vi "RW Cutoff Array.vi"(0 "Refnum In":T1, 2 "Read (F)":bool, 7 "CutoffArray In":cluster{"MidCutoff":dbl, "CloseCutoff":dbl}[](array[cluster]), 11 "Error In":errorcluster) -> (4 "Refnum Out":T1, 8 "CutoffArray Out":cluster{"MidCutoff":dbl, "CloseCutoff":dbl}[](array[cluster]), 15 "Error Out":errorcluster)   [LabVIEW 2013]
uses:
  <vilib>/Utility/config.llb/Config Data RefNum.ctl
  <vilib>/Utility/config.llb/Write Key (Double).vi
  <vilib>/Utility/config.llb/Read Key (Double).vi
  <vilib>/Utility/config.llb/NI_LVConfig.lvlib
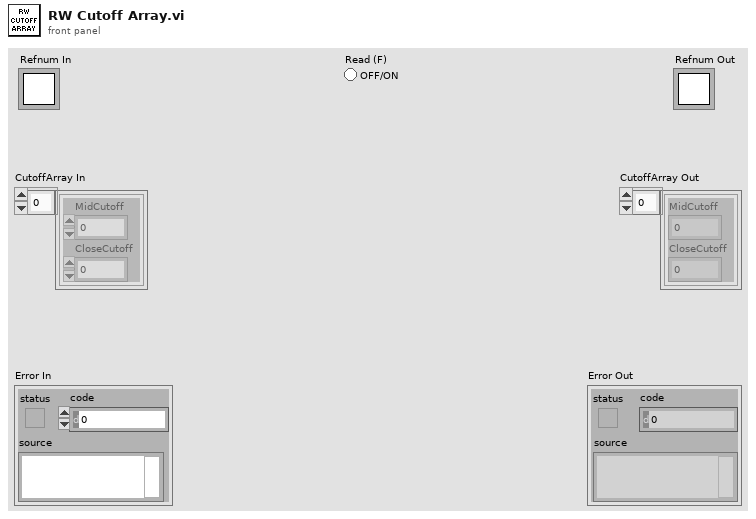
[diagram p1: front panel]
types:
  T1 = typedef "NI_LVConfig.lvlib/Config Data RefNum.ctl" = refnum<k1>
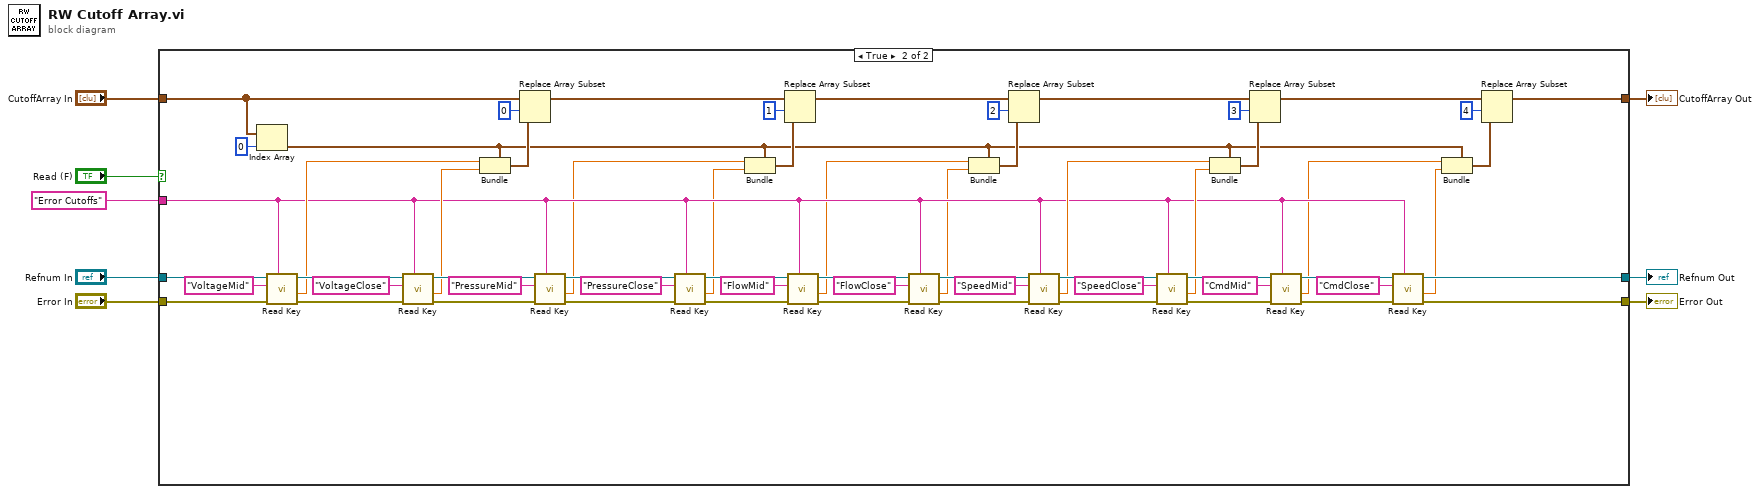
[diagram p0: block diagram]
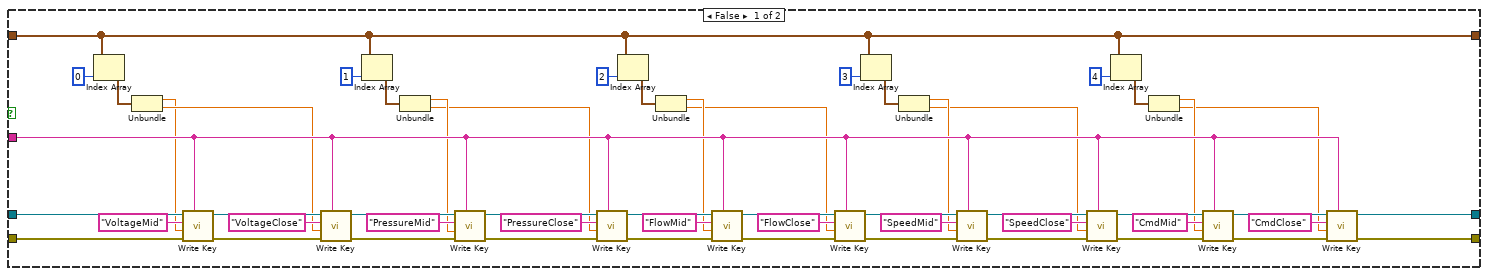
[diagram p2: hidden frame]
diagram:
  n1 = case shown="True" "Read (F)" {
    tunnel: "Error In" -> [w62 w122]
    tunnel: [w25 w89] -> w7
    tunnel: "Refnum In" -> [w53 w123]
    tunnel: [w26 w90] -> w4
    tunnel: "Error Cutoffs" ("section") -> [w24 w78]
    tunnel: "CutoffArray In" -> [w19 w104]
    tunnel: [w19 w70] -> w1
    frame False {
      n2 = Index Array(array=w19, index=0) -> (element=w44:cluster{"MidCutoff":dbl, "CloseCutoff":dbl})
      n3 = Unbundle(w44) -> ("MidCutoff"=w17:dbl, "CloseCutoff"=w18:dbl)
      n4 = call-poly <vilib>:"Write Key.vi"("section"=w24, "error in (no error)"=w62, "value"=w17, "key"="VoltageMid", "refnum"=w53) -> ("error out"=w61:errorcluster, "refnum out"=w52:T1)  [unwired: 4 in, 1 out]
      n5 = call-poly <vilib>:"Write Key.vi"("section"=w24, "error in (no error)"=w61, "value"=w18, "key"="VoltageClose", "refnum"=w52) -> ("error out"=w60:errorcluster, "refnum out"=w51:T1)  [unwired: 4 in, 1 out]
      n6 = Index Array(array=w19, index=1) -> (element=w41:cluster{"MidCutoff":dbl, "CloseCutoff":dbl})
      n7 = Unbundle(w41) -> ("MidCutoff"=w16:dbl, "CloseCutoff"=w15:dbl)
      n8 = call-poly <vilib>:"Write Key.vi"("section"=w24, "error in (no error)"=w60, "value"=w16, "key"="PressureMid", "refnum"=w51) -> ("error out"=w59:errorcluster, "refnum out"=w50:T1)  [unwired: 4 in, 1 out]
      n9 = call-poly <vilib>:"Write Key.vi"("section"=w24, "error in (no error)"=w59, "value"=w15, "key"="PressureClose", "refnum"=w50) -> ("error out"=w58:errorcluster, "refnum out"=w49:T1)  [unwired: 4 in, 1 out]
      n10 = Index Array(array=w19, index=2) -> (element=w40:cluster{"MidCutoff":dbl, "CloseCutoff":dbl})
      n11 = Unbundle(w40) -> ("MidCutoff"=w14:dbl, "CloseCutoff"=w13:dbl)
      n12 = call-poly <vilib>:"Write Key.vi"("section"=w24, "error in (no error)"=w58, "value"=w14, "key"="FlowMid", "refnum"=w49) -> ("error out"=w57:errorcluster, "refnum out"=w48:T1)  [unwired: 4 in, 1 out]
      n13 = call-poly <vilib>:"Write Key.vi"("section"=w24, "error in (no error)"=w57, "value"=w13, "key"="FlowClose", "refnum"=w48) -> ("error out"=w56:errorcluster, "refnum out"=w47:T1)  [unwired: 4 in, 1 out]
      n14 = Index Array(array=w19, index=3) -> (element=w22:cluster{"MidCutoff":dbl, "CloseCutoff":dbl})
      n15 = Unbundle(w22) -> ("MidCutoff"=w12:dbl, "CloseCutoff"=w11:dbl)
      n16 = call-poly <vilib>:"Write Key.vi"("section"=w24, "error in (no error)"=w56, "value"=w12, "key"="SpeedMid", "refnum"=w47) -> ("error out"=w55:errorcluster, "refnum out"=w46:T1)  [unwired: 4 in, 1 out]
      n17 = call-poly <vilib>:"Write Key.vi"("section"=w24, "error in (no error)"=w55, "value"=w11, "key"="SpeedClose", "refnum"=w46) -> ("error out"=w54:errorcluster, "refnum out"=w45:T1)  [unwired: 4 in, 1 out]
      n18 = Index Array(array=w19, index=4) -> (element=w21:cluster{"MidCutoff":dbl, "CloseCutoff":dbl})
      n19 = Unbundle(w21) -> ("MidCutoff"=w10:dbl, "CloseCutoff"=w9:dbl)
      n20 = call-poly <vilib>:"Write Key.vi"("section"=w24, "error in (no error)"=w54, "value"=w10, "key"="CmdMid", "refnum"=w45) -> ("error out"=w28:errorcluster, "refnum out"=w27:T1)  [unwired: 4 in, 1 out]
      n21 = call-poly <vilib>:"Write Key.vi"("section"=w24, "error in (no error)"=w28, "value"=w9, "key"="CmdClose", "refnum"=w27) -> ("error out"=w25:errorcluster, "refnum out"=w26:T1)  [unwired: 4 in, 1 out]
    }
    frame True {
      n22 = Index Array(array=w104, index=0) -> (element=w69:cluster{"MidCutoff":dbl, "CloseCutoff":dbl})
      n23 = call-poly <vilib>:"Read Key.vi"("section"=w78, "error in (no error)"=w122, "key"="VoltageMid", "refnum"=w123) -> ("error out"=w106:errorcluster, "value"=w93:dbl, "refnum out"=w121:T1)  [unwired: 4 in, 1 out]
      n24 = call-poly <vilib>:"Read Key.vi"("section"=w78, "error in (no error)"=w106, "key"="VoltageClose", "refnum"=w121) -> ("error out"=w107:errorcluster, "value"=w94:dbl, "refnum out"=w120:T1)  [unwired: 4 in, 1 out]
      n25 = Bundle(cluster=w69, "MidCutoff"=w93, "CloseCutoff"=w94) -> (w102:cluster{"MidCutoff":dbl, "CloseCutoff":dbl})
      n26 = Replace Array Subset(array=w104, new element=w102, index=0) -> (w73:cluster{"MidCutoff":dbl, "CloseCutoff":dbl}[])
      n27 = call-poly <vilib>:"Read Key.vi"("section"=w78, "error in (no error)"=w107, "key"="PressureMid", "refnum"=w120) -> ("error out"=w108:errorcluster, "value"=w68:dbl, "refnum out"=w119:T1)  [unwired: 4 in, 1 out]
      n28 = call-poly <vilib>:"Read Key.vi"("section"=w78, "error in (no error)"=w108, "key"="PressureClose", "refnum"=w119) -> ("error out"=w109:errorcluster, "value"=w67:dbl, "refnum out"=w118:T1)  [unwired: 4 in, 1 out]
      n29 = Bundle(cluster=w69, "MidCutoff"=w68, "CloseCutoff"=w67) -> (w74:cluster{"MidCutoff":dbl, "CloseCutoff":dbl})
      n30 = Replace Array Subset(array=w73, new element=w74, index=1) -> (w72:cluster{"MidCutoff":dbl, "CloseCutoff":dbl}[])
      n31 = call-poly <vilib>:"Read Key.vi"("section"=w78, "error in (no error)"=w109, "key"="FlowMid", "refnum"=w118) -> ("error out"=w110:errorcluster, "value"=w66:dbl, "refnum out"=w117:T1)  [unwired: 4 in, 1 out]
      n32 = call-poly <vilib>:"Read Key.vi"("section"=w78, "error in (no error)"=w110, "key"="FlowClose", "refnum"=w117) -> ("error out"=w111:errorcluster, "value"=w65:dbl, "refnum out"=w116:T1)  [unwired: 4 in, 1 out]
      n33 = Bundle(cluster=w69, "MidCutoff"=w66, "CloseCutoff"=w65) -> (w101:cluster{"MidCutoff":dbl, "CloseCutoff":dbl})
      n34 = Replace Array Subset(array=w72, new element=w101, index=2) -> (w103:cluster{"MidCutoff":dbl, "CloseCutoff":dbl}[])
      n35 = call-poly <vilib>:"Read Key.vi"("section"=w78, "error in (no error)"=w111, "key"="SpeedMid", "refnum"=w116) -> ("error out"=w112:errorcluster, "value"=w95:dbl, "refnum out"=w115:T1)  [unwired: 4 in, 1 out]
      n36 = call-poly <vilib>:"Read Key.vi"("section"=w78, "error in (no error)"=w112, "key"="SpeedClose", "refnum"=w115) -> ("error out"=w113:errorcluster, "value"=w96:dbl, "refnum out"=w114:T1)  [unwired: 4 in, 1 out]
      n37 = Bundle(cluster=w69, "MidCutoff"=w95, "CloseCutoff"=w96) -> (w100:cluster{"MidCutoff":dbl, "CloseCutoff":dbl})
      n38 = Replace Array Subset(array=w103, new element=w100, index=3) -> (w71:cluster{"MidCutoff":dbl, "CloseCutoff":dbl}[])
      n39 = call-poly <vilib>:"Read Key.vi"("section"=w78, "error in (no error)"=w113, "key"="CmdMid", "refnum"=w114) -> ("error out"=w92:errorcluster, "value"=w64:dbl, "refnum out"=w91:T1)  [unwired: 4 in, 1 out]
      n40 = call-poly <vilib>:"Read Key.vi"("section"=w78, "error in (no error)"=w92, "key"="CmdClose", "refnum"=w91) -> ("error out"=w89:errorcluster, "value"=w63:dbl, "refnum out"=w90:T1)  [unwired: 4 in, 1 out]
      n41 = Bundle(cluster=w69, "MidCutoff"=w64, "CloseCutoff"=w63) -> (w76:cluster{"MidCutoff":dbl, "CloseCutoff":dbl})
      n42 = Replace Array Subset(array=w71, new element=w76, index=4) -> (w70:cluster{"MidCutoff":dbl, "CloseCutoff":dbl}[])
    }
  }
  "Refnum Out" <- w4
  "Error Out" <- w7
  "CutoffArray Out" <- w1
